vi "IEEE 1588-2008 Find Clocks (modified).vi"(8 "Clock Id to Verify":string="00-80-2F-FF-FE-12-6A-FD:1") -> (0 "Synced?":bool)   [LabVIEW 2014]
uses:
  <vilib>/nisyscfg/Initialize (Control).vi
  <vilib>/nisyscfg/Find Hardware.vi
  <vilib>/nisyscfg/Close (Hardware).vi
  <vilib>/nisyscfg/Close (System).vi
  <vilib>/nisyscfg/nisyscfg.lvlib
  <resource>/objmgr/niflexriosae.rc
panel:
  out "error out":errorcluster
  in  "error in (no error)":errorcluster
  in  "System (defaults to localhost)":refnum<k21>="localhost"
  out "Multicolumn Listbox":i32(listbox)
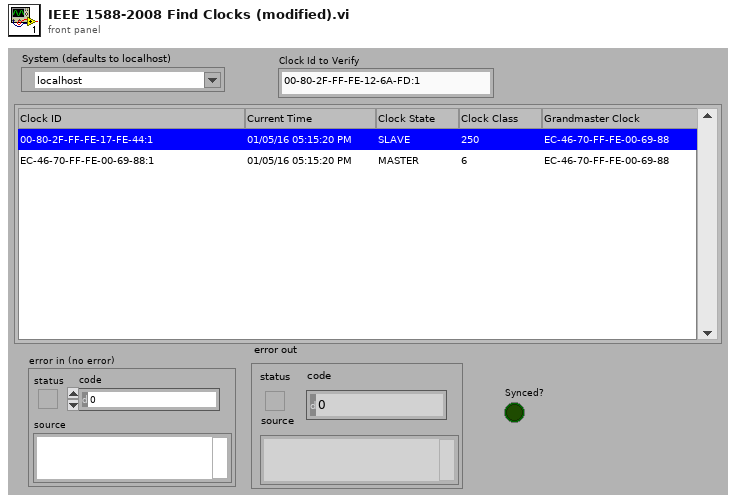
[diagram p1: front panel]
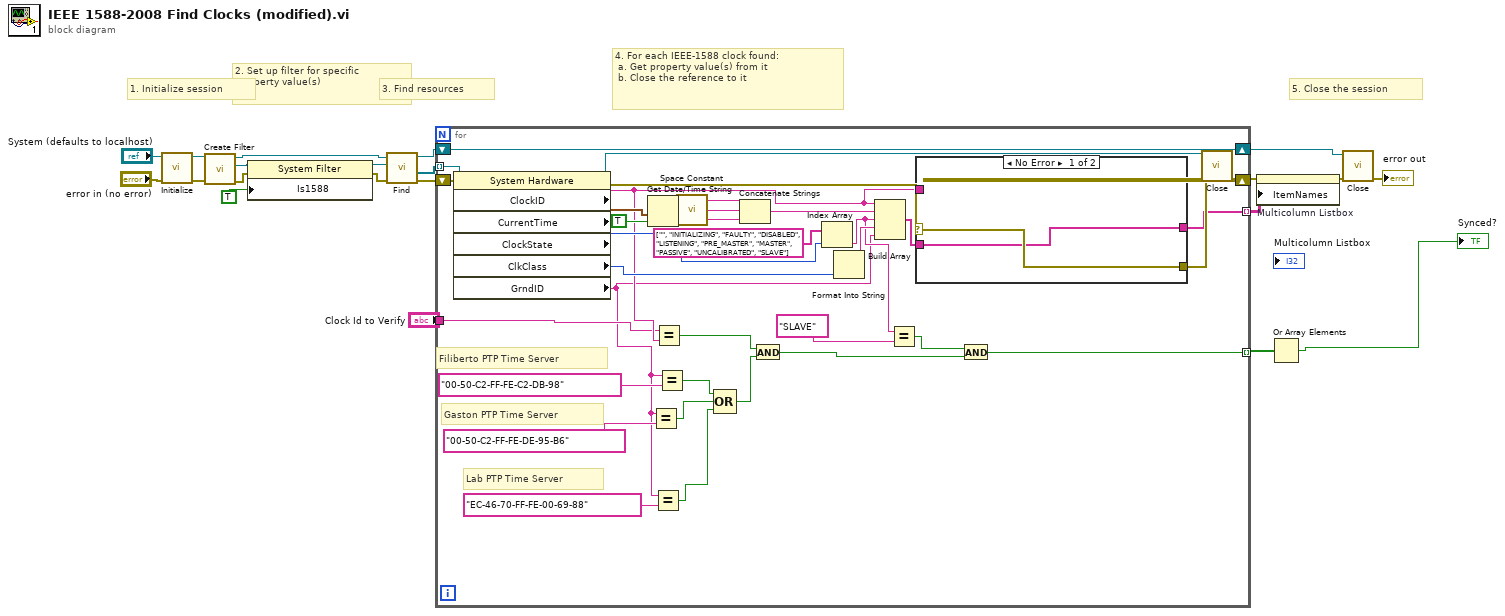
[diagram p0: block diagram]
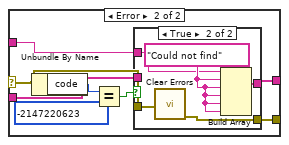
[diagram p2: hidden frame]
diagram:
  # "2. Set up filter for specific \n property value(s)"
  # "3. Find resources"
  # "5. Close the session"
  # "4. For each IEEE-1588 clock found:\n a. Get property value(s) from it\n b. Close the reference to it"
  # "1. Initialize session"
  n1 = call-poly <vilib>:"Initialize.vi"("error in (no error)"="error in (no error)", "Target (localhost)"="System (defaults to localhost)") -> ("error out"=w12:errorcluster, "Session out"=w13:refnum<k21>)  [unwired: 7 in, 1 out]
  n2 = call <vilib>:"Create Filter.vi"("error in (no error)"=w12, "Session in"=w13) -> ("error out"=w10:errorcluster, "Filter out"=w7:refnum<k20>, "Session out"=w14:refnum<k21>)  [unwired: 7 in]
  n3 = property class="System Filter"(reference=w7, error in=w10, "Is1588"=TRUE ("Item Specific:Is 1588")) -> (reference out=w8:refnum<k20>, error out=w9:errorcluster)
  n4 = call-poly <vilib>:"Find.vi"("error in (no error)"=w9, "Filter in"=w8, "Session in"=w14) -> ("error out"=w21:errorcluster, "Resources out"=w20:refnum<k20>[], "Session out"=w19:refnum<k21>)  [unwired: 5 in, 1 out]
  n5 = for {
    shift-right: [w51] -> w18
    shift-left: w21 -> [w47]
    tunnel: w20 -> [w45] mode=indexing
    tunnel: [w39] -> w4 mode=indexing
    shift-right: [w52] -> w17
    shift-left: w19 -> [w52]
    tunnel: [w33] -> w2 mode=indexing
    tunnel: "Clock Id to Verify" -> [w32]
    # "Gaston PTP Time Server"
    # "Filiberto PTP Time Server"
    # "Lab PTP Time Server"
    n6 = property class="System Hardware"(reference=w45, error in=w47) -> (reference out=w46:refnum<k20>, error out=w40:errorcluster, "ClockID"=w37:string, "CurrentTime"=w44:timestamp, "ClockState"=w43:i32, "ClkClass"=w42:u32, "GrndID"=w24:string)
    n7 = Get Date/Time String(seconds (now)=w44, want seconds? (F)=TRUE) -> (date string=w54:string, time string=w50:string)  [unwired: 1 in]
    n8 = Equal?(x=w24, y="00-50-C2-FF-FE-DE-95-B6") -> (x = y?=w28:bool)
    n9 = Equal?(x=w24, y="EC-46-70-FF-FE-00-69-88") -> (x = y?=w22:bool)
    n10 = Equal?(x=w32, y=w37) -> (x = y?=w26:bool)
    n11 = Equal?(x=w24, y="00-50-C2-FF-FE-C2-DB-98") -> (x = y?=w29:bool)
    n12 = call <vilib>:"Space Constant.vi"() -> ("String"=w49:string)
    n13 = Compound Arithmetic op=OR(w29, w28, w22) -> (w27:bool)
    n14 = Concatenate Strings(w54, w49, w50) -> (w53:string)
    n15 = And(x=w26, y=w27) -> (x .and. y?=w25:bool)
    n16 = Index Array(array=string[] ["", "INITIALIZING", "FAULTY", "DISABLED", "LISTENING", "PRE_MASTER", "MASTER", "PASSIVE", "UNCALIBRATED", "SLAVE"], index=w43) -> (element=w36:string)
    n17 = Format Into String(w42) -> (resulting string=w48:string)  [unwired: 3 in, 1 out]
    n18 = Build Array(w37, w53, w36, w48, w24) -> (w38:string[])
    n19 = Equal?(x=w36, y="SLAVE") -> (x = y?=w34:bool)
    n20 = case shown="No Error" w40 {
      selector: w40 -> [w58 w63]
      tunnel: [w58 w59] -> w41
      tunnel: w38 -> [w57 w62]
      tunnel: [w57 w61] -> w39
      tunnel: w37 -> [_ w60]
      frame No Error {
      }
      frame Error {
        n21 = Unbundle By Name(w63) -> ("code"=w66:i32)
        n22 = Equal?(x=w66, y=-2147220623) -> (x = y?=w64:bool)
        n23 = case shown="True" w64 {
          tunnel: w63 -> [w68 w72]
          tunnel: [w68 w73] -> w59
          tunnel: w62 -> [w67 _]
          tunnel: [w67 w71] -> w61
          tunnel: w60 -> [_ w69]
          frame False {
          }
          frame True {
            w70 = "Could not find"
            n24 = call <vilib>:"Clear Errors.vi"("error in (no error)"=w72) -> ("error out"=w73:errorcluster)  [unwired: 5 in, 1 out]
            n25 = Build Array(w69, w70, w70, w70, w70, w70) -> (w71:string[])
          }
        }
      }
    }
    n26 = And(x=w34, y=w25) -> (x .and. y?=w33:bool)
    n27 = call-poly <vilib>:"Close.vi"("error in (no error)"=w41, "Resource in"=w46) -> ("error out"=w51:errorcluster)  [unwired: 9 in]
  }
  n28 = property on="Multicolumn Listbox" class="MCListbox (strict)"(error in=w18, "ItemNames"=w4) -> (error out=w16:errorcluster)  [unwired: 1 in, 1 out]
  n29 = Or Array Elements(Boolean array=w2) -> (logical OR=→"Synced?":bool)
  n30 = call-poly <vilib>:"Close.vi"("error in (no error)"=w16, "Session in"=w17) -> ("error out"=→"error out":errorcluster)  [unwired: 9 in]
